vi "Map Channels.vi"   [LabVIEW 2016, in "System Mapping Tool.lvlib"]
uses:
  System Mapping Tool.lvlib
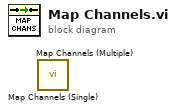
[diagram p0: block diagram]
diagram:
  n1 = call "Map Channels (Single).vi"() -> ()  [unwired: 11 in, 1 out]
  n2 = call "Map Channels (Multiple).vi"() -> ()  [unwired: 11 in, 1 out]
